vi "Knob Fill (Two-Way).vi"(8 "Default Value":dbl, 9 "Value":dbl, 10 "Maximum":dbl, 11 "Minimum":dbl) -> (3 "Marker Values":cluster{"Value":dbl, "Color Box":u32}[](array[cluster]))   [LabVIEW 2019, in "User Interface.lvlib"]
doc: "Logic for a two-way marker fill, from default to min, or from default to max."
uses:
  User Interface.lvlib
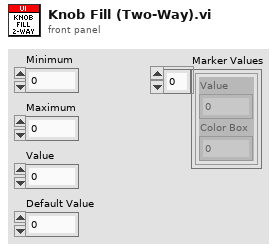
[diagram p1: front panel]
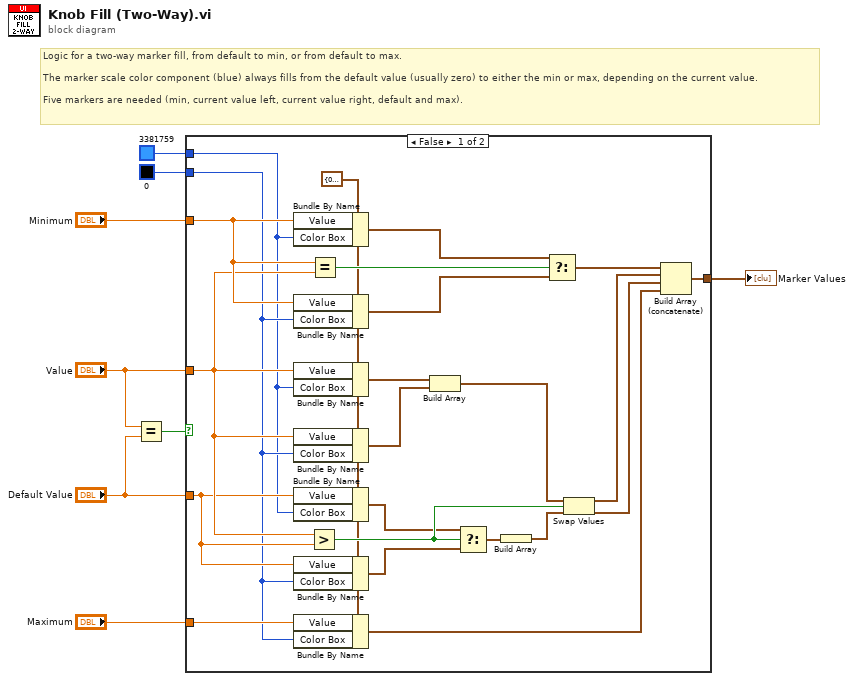
[diagram p0: block diagram]
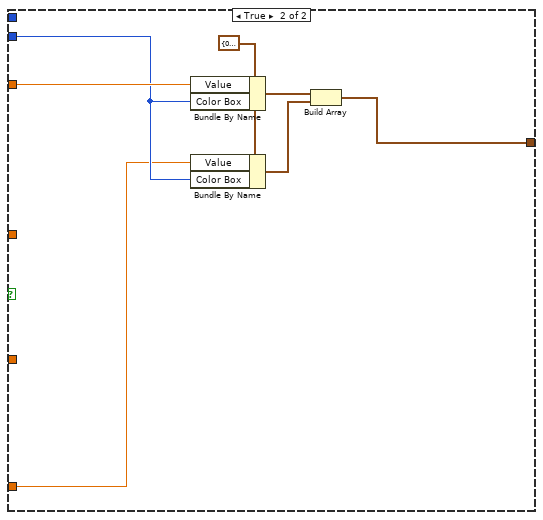
[diagram p2: hidden frame]
diagram:
  # "Logic for a two-way marker fill, from default to min, or from default to max.\n\nThe marker scale color component (blue) always fills from the default value (usually zero) to either the min or max, depending on the current value.\n\nFive markers are needed (min, current value left, current value right, default and max)."
  n1 = Equal?(x="Value", y="Default Value") -> (x = y?=w1:bool)
  n2 = case shown="False" w1 {
    tunnel: [w30 w32] -> w8
    tunnel: "Minimum" -> [w14 w38]
    tunnel: "Maximum" -> [w13 w36]
    tunnel: "Value" -> [w12 _]
    tunnel: "Default Value" -> [w11 _]
    tunnel: u32 0 ("Color Box") -> [w10 w37]
    tunnel: u32 3381759 ("Color Box") -> [w9 _]
    frame False {
      w15 = cluster{"Value":dbl, "Color Box":u32} {"Value"=0.0, "Color Box"=0}
      n3 = Bundle By Name(cluster=w15, "Value"=w14, "Color Box"=w9) -> (w20:cluster{"Value":dbl, "Color Box":u32})
      n4 = Bundle By Name(cluster=w15, "Value"=w14, "Color Box"=w10) -> (w19:cluster{"Value":dbl, "Color Box":u32})
      n5 = Bundle By Name(cluster=w15, "Value"=w12, "Color Box"=w9) -> (w26:cluster{"Value":dbl, "Color Box":u32})
      n6 = Bundle By Name(cluster=w15, "Value"=w12, "Color Box"=w10) -> (w25:cluster{"Value":dbl, "Color Box":u32})
      n7 = Bundle By Name(cluster=w15, "Value"=w11, "Color Box"=w9) -> (w17:cluster{"Value":dbl, "Color Box":u32})
      n8 = Bundle By Name(cluster=w15, "Value"=w11, "Color Box"=w10) -> (w16:cluster{"Value":dbl, "Color Box":u32})
      n9 = Bundle By Name(cluster=w15, "Value"=w13, "Color Box"=w10) -> (w29:cluster{"Value":dbl, "Color Box":u32})
      n10 = Greater?(x=w12, y=w11) -> (0:w18:bool)
      n11 = Equal?(x=w14, y=w12) -> (x = y?=w31:bool)
      n12 = Build Array(w26, w25) -> (w24:cluster{"Value":dbl, "Color Box":u32}[])
      n13 = Select(t=w17, s=w18, f=w16) -> (s? t:f=w27:cluster{"Value":dbl, "Color Box":u32})
      n14 = Build Array(w27) -> (w21:cluster{"Value":dbl, "Color Box":u32}[])
      n15 = Select(t=w20, s=w31, f=w19) -> (s? t:f=w28:cluster{"Value":dbl, "Color Box":u32})
      n16 = Swap Values(12:w24, 13:w18, 14:w21) -> (1:w23:cluster{"Value":dbl, "Color Box":u32}[], 3:w22:cluster{"Value":dbl, "Color Box":u32}[])
      n17 = Build Array (concatenate)(w28, w23, w22, w29) -> (w30:cluster{"Value":dbl, "Color Box":u32}[])
    }
    frame True {
      w34 = cluster{"Value":dbl, "Color Box":u32} {"Value"=0.0, "Color Box"=0}
      n18 = Bundle By Name(cluster=w34, "Value"=w38, "Color Box"=w37) -> (w35:cluster{"Value":dbl, "Color Box":u32})
      n19 = Bundle By Name(cluster=w34, "Value"=w36, "Color Box"=w37) -> (w33:cluster{"Value":dbl, "Color Box":u32})
      n20 = Build Array(w35, w33) -> (w32:cluster{"Value":dbl, "Color Box":u32}[])
    }
  }
  "Marker Values" <- w8
